vi "setResolution.vi"(8 "error in (no error)":errorcluster, 11 "reference in":refnum<class "GUI Controller.lvclass">) -> (0 "error out":errorcluster, 3 "reference out":refnum<class "GUI Controller.lvclass">)   [LabVIEW 2016, in "GUI Controller.lvclass"]
uses:
  GUI Controller.lvclass
  USER32.DLL
  Project Panels_class/Project Panels.lvclass
panel:
  out "screenHeight":i32
  out "screenWidth":i32
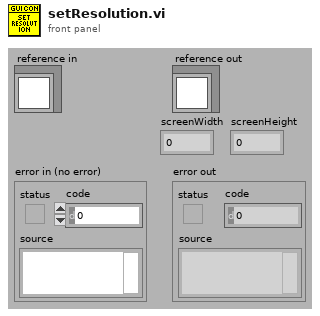
[diagram p1: front panel]
types:
  T1 = typedef "GUI Controller.lvclass/ObjectAttributesRef.ctl" = refnum<data-value>
  T2 = typedef "GUI Controller.lvclass/ObjectAttributes.ctl" = cluster{"MyAttribute":dbl, "state":T3, "project_panels_ref":refnum<class "Project Panels.lvclass">, "items_controller_ref":refnum<class "Items Controller.lvclass">, "notification_controller_ref":refnum<class "Notification Controller.lvclass">, "partstracking_controller_ref":refnum<class "PartsTracking Controller.lvclass">, "file_controller_ref":refnum<class "File Controller.lvclass">, "low_resolution?":bool, "run_python?":bool}
  T3 = typedef "GUI Controller.lvclass/state.ctl" = enum16{"initiate", "checkNotificationItems", "checkNotificationTracking", "operate", "updateFromFile", "stop"}
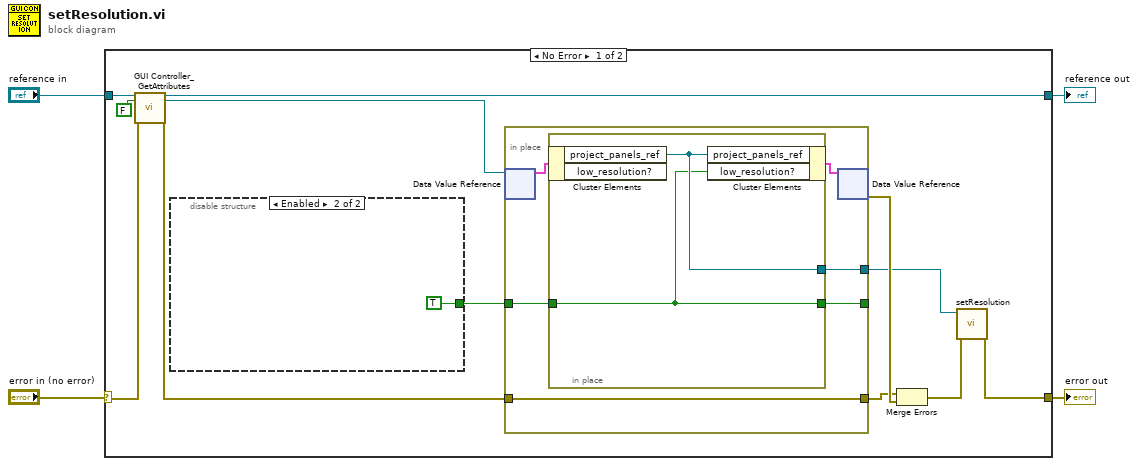
[diagram p0: block diagram]
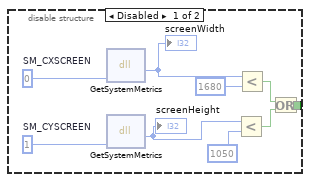
[diagram p2: hidden frame]
diagram:
  n1 = case shown="No Error" "error in (no error)" {
    selector: "error in (no error)" -> [w12 w35]
    tunnel: [w7 w35] -> w3
    tunnel: [w10 w34] -> w1
    tunnel: "reference in" -> [w14 w34]
    frame No Error {
      n2 = call "GUI Controller_GetAttributes.vi"("reference in"=w14, "return data? (T)"=FALSE, "error in (no error)"=w12) -> ("reference out"=w10:refnum<class "GUI Controller.lvclass">, "attributes ref"=w9:T1, "error out"=w11:errorcluster)  [unwired: 13 in, 1 out]
      n3 = disable-structure shown="Enabled" {
        disable-tunnel: [_ TRUE] -> w5
        frame Disabled {
          w23 = 1  # SM_CYSCREEN
          w24 = 0  # SM_CXSCREEN
          n4 = dll-call lib="USER32.DLL" fn="GetSystemMetrics"("parameter"=w24) -> ("screenWidth"=w22:i32)  [unwired: 4 in, 2 out]
          "screenWidth" <- w22
          n5 = dll-call lib="USER32.DLL" fn="GetSystemMetrics"("parameter"=w23) -> ("screenHeight"=w20:i32)  [unwired: 4 in, 2 out]
          "screenHeight" <- w20
          n6 = Less?(x=w20, y=1050) -> (x < y?=w17:bool)
          n7 = Less?(x=w22, y=1680) -> (x < y?=w18:bool)
          n8 = Or(x=w18, y=w17) -> ()  [unwired: 1 out]
        }
        frame Enabled {
        }
      }
      n9 = in-place {
        in-place-border: w11 -> [w29]
        in-place-border: [w29] -> w15
        in-place-border: w5 -> [w28]
        in-place-border: [w27] -> w6
        in-place-border: [w26] -> _
        n10 = in-place-dvr #1(w9) -> (w30:T2)  [unwired: 1 out]
        n11 = in-place {
          in-place-border: w28 -> [w32]
          in-place-border: [w33] -> w27
          in-place-border: [w32] -> w26
          n12 = in-place-cluster #2(w30) -> ("project_panels_ref"=w33:refnum<class "Project Panels.lvclass">)  [unwired: 1 out]
          n13 = in-place-cluster #2("project_panels_ref"=w33, "low_resolution?"=w32) -> (w31:T2)
        }
        n14 = in-place-dvr #1(w31) -> (w16:errorcluster)  [unwired: 1 out]
      }
      n15 = Merge Errors(w15, w16) -> (w8:errorcluster)
      n16 = call "setResolution.vi"("error in (no error)"=w8, "reference in"=w6) -> ("error out"=w7:errorcluster)  [unwired: 8 in, 1 out]
    }
    frame Error {
    }
  }
  "error out" <- w3
  "reference out" <- w1
